vi "Init_Test.vi"(8 "error in (no error)":errorcluster caption="entrée d'erreur (pas d'erreur)", 11 "Test (Default) en entrée":refnum<class "Sequencer_With_Database.lvclass">) -> (0 "error out":errorcluster caption="sortie d'erreur", 3 "Test (Default) en sortie":refnum<class "Sequencer_With_Database.lvclass">)   [LabVIEW 2020, in "Library Core.lvlib" / "Sequencer_With_Database.lvclass"]
uses:
  Sequencer_With_Database.lvclass
  C:/Users/ngarcin/OneDrive - Altyor/Standard TB/Class/Sequencer/Sequencer (Default)/Sequencer (Default).lvclass
  Commun VI/TypeDef/Actor Type.ctl
  Sequencer (Default)/Sequencer (Default).lvclass
  Sequencer_With_Database.lvclass/Sequencer_With_Database.ctl
  Commun VI/Library Commun.lvlib
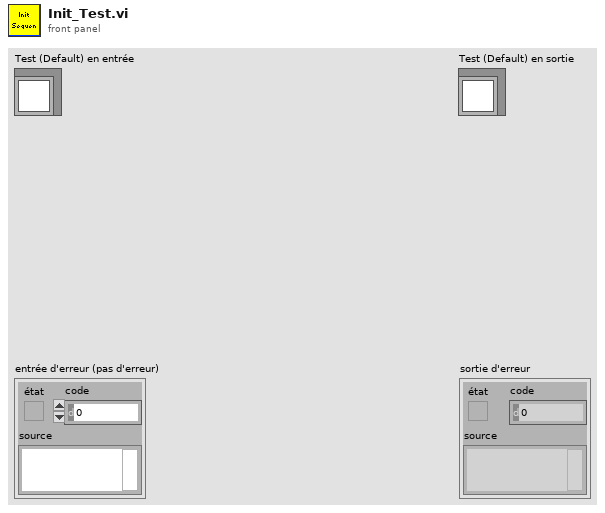
[diagram p1: front panel]
types:
  T1 = typedef "Library Commun.lvlib/Actor Type.ctl" = enum16{"Default", "Firebase", "Database"}
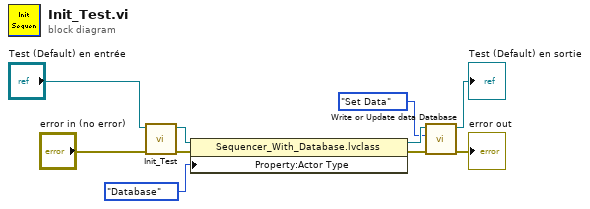
[diagram p0: block diagram]
diagram:
  n1 = call-parent "Init_Test.vi"("error in (no error)"="error in (no error)", "Test (Default) en entrée"="Test (Default) en entrée") -> ("error out"=w4:errorcluster, "Test (Default) en sortie"=w6:refnum<class "Sequencer_With_Database.lvclass">)  [unwired: 8 in]
  n2 = property class="Sequencer_With_Database.lvclass"(reference=w6, error in=w4, "Property:Actor Type"=Actor_Type."Database" ("Actor Type")) -> (reference out=w2:refnum<class "Sequencer_With_Database.lvclass">, error out=w3:errorcluster)
  n3 = call-dynamic "Write or Update data Database.vi"("error in (no error)"=w3, "Function"=enum16{"Set Data", "Update Data"}."Set Data", "Sequencer IN"=w2) -> ("error out"=→"error out":errorcluster, "Sequencer Out"=→"Test (Default) en sortie":refnum<class "Sequencer_With_Database.lvclass">)  [unwired: 7 in]
